vi "Get Language of file.vi"(11 "FileName":string) -> (3 "substring before match":string)   [LabVIEW 2012]
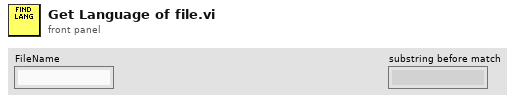
[diagram p1: front panel]
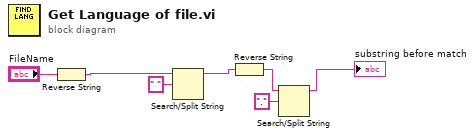
[diagram p0: block diagram]
diagram:
  n1 = Reverse String(1:"FileName") -> (0:w7:string)
  n2 = Search/Split String(string=w7, search string/char (-)=" ") -> (substring before match=w5:string)  [unwired: 1 in, 2 out]
  n3 = Reverse String(1:w5) -> (0:w4:string)
  n4 = Search/Split String(string=w4, search string/char (-)=".") -> (substring before match=→"substring before match":string)  [unwired: 1 in, 2 out]
